vi "SearchForTicket.vi"(0 "Licence":string, 3 "error in":errorcluster, 4 "Database":string[][](array[string])) -> (7 "TicketDuration":i32, 10 "error out":errorcluster)   [LabVIEW 2019]
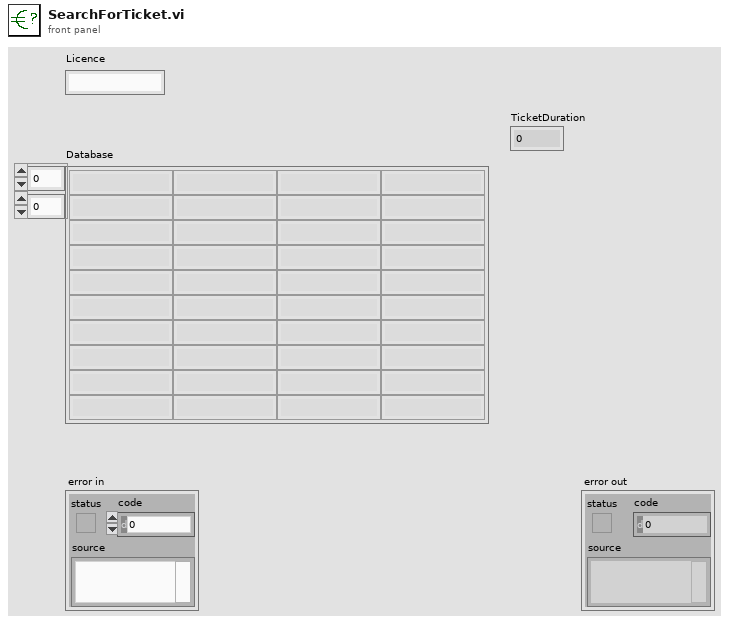
[diagram p1: front panel]
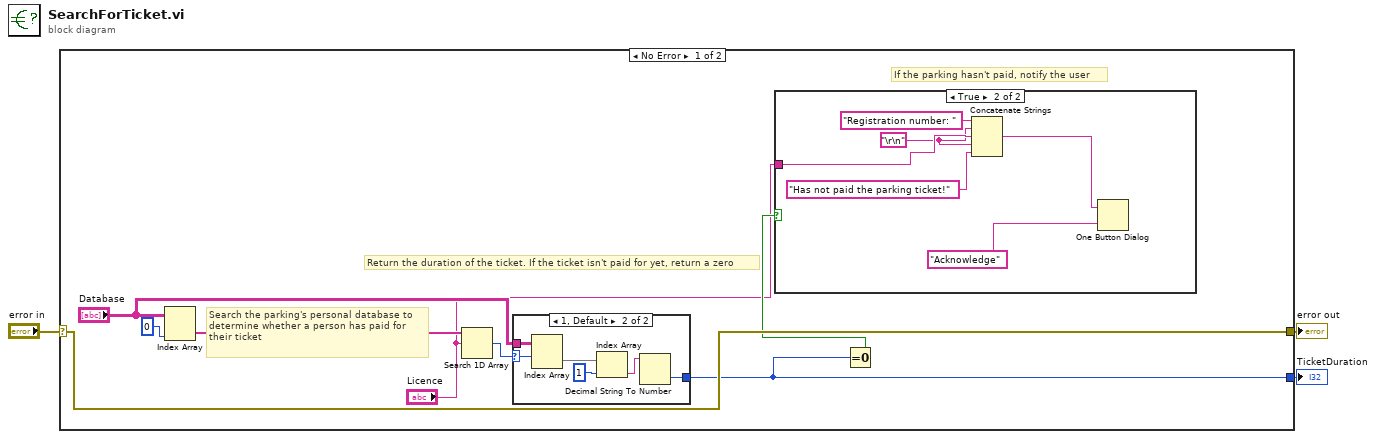
[diagram p0: block diagram]
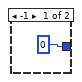
[diagram p3: hidden frame]
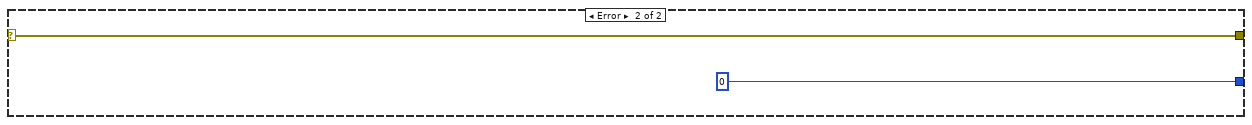
[diagram p4: hidden frame]
diagram:
  n1 = case shown="No Error" "error in" {
    selector: "error in" -> [w8 w26]
    tunnel: [w8 w26] -> w2
    tunnel: [w6 0] -> w1
    frame No Error {
      # "If the parking hasn't paid, notify the user"
      # "Return the duration of the ticket. If the ticket isn't paid for yet, return a zero"
      # "Search the parking's personal database to\ndetermine whether a person has paid for\ntheir ticket"
      n2 = Index Array(array="Database", index (col)=0 ("disabled index (col)")) -> (element=w11:string[])  [unwired: 1 in]
      n3 = Search 1D Array(1D array=w11, element="Licence") -> (index of element=w9:i32)  [unwired: 1 in]
      n4 = case shown="1, Default" w9 {
        selector: w9 -> [_ w22]
        tunnel: "Database" -> [_ w23]
        tunnel: [0 w19] -> w6
        frame -1 {
        }
        frame 1, Default {
          n5 = Index Array(array=w23, index (row)=w22) -> (element=w21:string[])  [unwired: 1 in]
          n6 = Index Array(array=w21, index=1) -> (element=w20:string)
          n7 = Decimal String To Number(string=w20) -> (number=w19:i32)  [unwired: 2 in, 1 out]
        }
      }
      n8 = Equal To 0?(x=w6) -> (x = 0?=w5:bool)
      n9 = case shown="True" w5 {
        tunnel: "Licence" -> [_ w15]
        frame False {
        }
        frame True {
          w14 = "\r\n"
          n10 = Concatenate Strings("Registration number: " ("string"), w14, w15, w14, "Has not paid the parking ticket!" ("message")) -> (w12:string)
          n11 = One Button Dialog(message=w12, button name ("OK")="Acknowledge") -> ()  [unwired: 1 out]
        }
      }
    }
    frame Error {
    }
  }
  "error out" <- w2
  "TicketDuration" <- w1
